vi "Start heating and stirring for an amount of time.vi"() -> ()   [LabVIEW 2018, in "Hei-End.lvlib"]
uses:
  <instrlib>/Hei-End/Hei-End.lvlib
  <vilib>/Instr/_visa.llb/VISA Configure Serial Port (Instr).vi
panel:
  in  "Temperature (C)":i16
  in  "Motor speed (50rpm)":i16=50
  out "Elapsed Time (s)":dbl
  in  "Stop":bool
  in  "Time Target (s)":dbl=1.0
  in  "VISA resource name":refnum<visa-resource-name>
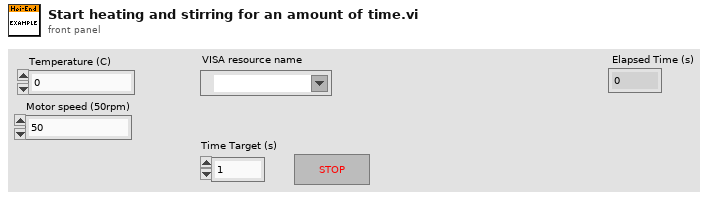
[diagram p1: front panel]
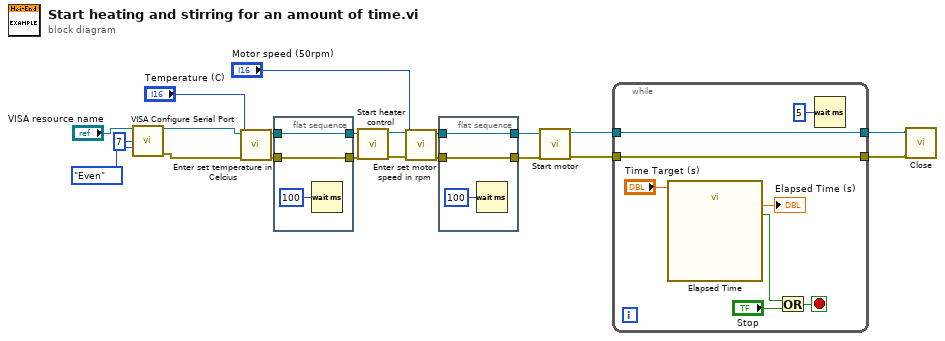
[diagram p0: block diagram]
diagram:
  n1 = call-poly "VISA Configure Serial Port"("VISA resource name"="VISA resource name", "data bits (8)"=u16 7, "parity (0:none)"=enum16{"None", "Odd", "Even", "Mark", "Space"}."Even") -> ("VISA resource name out"=w11:refnum<visa-resource-name>, "error out"=w12:errorcluster)  [unwired: 11 in]
  n2 = call <instrlib>:"Enter set temperature in Celcius.vi"("error in (no error)"=w12, "Temperature (C)"="Temperature (C)", "VISA resource name"=w11) -> ("error out"=w6:errorcluster, "VISA resource name out"=w8:refnum<visa-resource-name>)  [unwired: 7 in]
  n3 = flat-sequence {
    tunnel: w8 -> [w24]
    tunnel: [w24] -> w7
    tunnel: w6 -> [w23]
    tunnel: [w23] -> w5
    frame #0 {
      n4 = Wait (ms)(milliseconds to wait=u32 100) -> ()  [unwired: 1 out]
    }
  }
  n5 = call <instrlib>:"Start heater control.vi"("error in (no error)"=w5, "VISA resource name"=w7) -> ("error out"=w19:errorcluster, "VISA resource name out"=w20:refnum<visa-resource-name>)  [unwired: 8 in]
  n6 = call <instrlib>:"Enter set motor speed in rpm.vi"("error in (no error)"=w19, "Motor speed (10rpm)"="Motor speed (50rpm)", "VISA resource name"=w20) -> ("error out"=w1:errorcluster, "VISA resource name out"=w2:refnum<visa-resource-name>)  [unwired: 7 in]
  n7 = flat-sequence {
    tunnel: w2 -> [w27]
    tunnel: [w27] -> w4
    tunnel: w1 -> [w26]
    tunnel: [w26] -> w3
    frame #0 {
      n8 = Wait (ms)(milliseconds to wait=u32 100) -> ()  [unwired: 1 out]
    }
  }
  n9 = call <instrlib>:"Start motor.vi"("error in (no error)"=w3, "VISA resource name"=w4) -> ("error out"=w16:errorcluster, "VISA resource name out"=w17:refnum<visa-resource-name>)  [unwired: 8 in]
  n10 = while {
    tunnel: w17 -> [w31]
    tunnel: w16 -> [w30]
    tunnel: [w31] -> w15
    tunnel: [w30] -> w14
    stop <- w34 stop-if-true
    n11 = call "Elapsed Time"("Time Target (s)"="Time Target (s)") -> ("Elapsed Time (s)"=→"Elapsed Time (s)":dbl, "Time has Elapsed"=w33:bool)  [unwired: 11 in, 6 out]
    n12 = Or(x=w33, y="Stop") -> (x .or. y?=w34:bool)
    n13 = Wait (ms)(milliseconds to wait=u32 5) -> ()  [unwired: 1 out]
  }
  n14 = call <instrlib>:"Close.vi"("error in (no error)"=w14, "VISA resource name"=w15) -> ()  [unwired: 9 in, 1 out]
